vi "Actor Teardown.vi"(10 "Error":errorcluster, 11 "Self Actor in":refnum<class "Self Actor.lvclass">) -> (0 "error out":errorcluster, 2 "Teardown?":bool, 3 "Self Actor out":refnum<class "Self Actor.lvclass">)   [LabVIEW 2021, in "jettl.lvlib" / "Self Actor.lvclass"]
uses:
  Self Actor.lvclass
  C:/git/jettl/src/LVCAM/LVCAM/Actor/Actor.lvclass
  Self Actor.lvclass/Self Actor.ctl
  Self Actor State/Self Actor State.lvclass
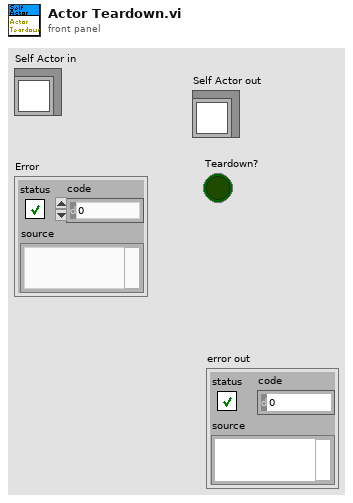
[diagram p1: front panel]
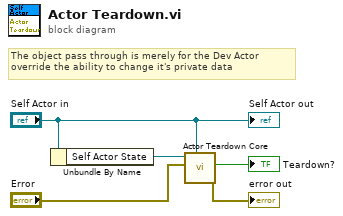
[diagram p0: block diagram]
diagram:
  # "The object pass through is merely for the Dev Actor override the ability to change it's private data"
  n1 = Unbundle By Name("Self Actor in") -> ("Self Actor State"=w5:refnum<class "Self Actor State.lvclass">)
  n2 = call-dynamic "Actor Teardown Core.vi"("Actor"="Self Actor in", "Error"="Error", "Self Actor State in"=w5) -> ("error out"=→"error out":errorcluster, "Teardown?"=→"Teardown?":bool)  [unwired: 7 in]
  "Self Actor out" <- "Self Actor in"
